vi "load_array_of_channels_xml.vi"(8 "error in":errorcluster, 11 "node in":refnum<k20>) -> (0 "error out":errorcluster, 2 "Array of DDS Channels (4)":T1=[{"Power"=FALSE, "Channel Parameters"={"Ref Clock Rate [kHz]"=1000.0, "Full Scale Output\nPower [dBm]"=0.0}, "RAM Enable"=FALSE, "RAM Dest Type"=0, "RAM Default"={"Frequency [MHz]"=0.0, "Amplitude [dBm]"=0.0, "Phase Offset [rad]"=0.0}, "Array of DDS Profiles (8)"=[], "description"=""}, {"Power"=FALSE, "Channel Parameters"={"Ref Clock Rate [kHz]"=1000.0, "Full Scale Output\nPower [dBm]"=0.0}, "RAM Enable"=FALSE, "RAM Dest Type"=0, "RAM Default"={"Frequency [MHz]"=0.0, "Amplitude [dBm]"=0.0, "Phase Offset [rad]"=0.0}, "Array of DDS Profiles (8)"=[], "description"=""}, {"Power"=FALSE, "Channel Parameters"={"Ref Clock Rate [kHz]"=1000.0, "Full Scale Output\nPower [dBm]"=0.0}, "RAM Enable"=FALSE, "RAM Dest Type"=0, "RAM Default"={"Frequency [MHz]"=0.0, "Amplitude [dBm]"=0.0, "Phase Offset [rad]"=0.0}, "Array of DDS Profiles (8)"=[], "description"=""}, {"Power"=FALSE, "Channel Parameters"={"Ref Clock Rate [kHz]"=1000.0, "Full Scale Output\nPower [dBm]"=0.0}, "RAM Enable"=FALSE, "RAM Dest Type"=0, "RAM Default"={"Frequency [MHz]"=0.0, "Amplitude [dBm]"=0.0, "Phase Offset [rad]"=0.0}, "Array of DDS Profiles (8)"=[], "description"=""}] {"Channel Parameters"."Ref Clock Rate [kHz]" min=0.0}, 3 "node":refnum<k20>)   [LabVIEW 2013, in "DDS.lvclass"]
doc: "Loads an array of DDS channels from xml. Expected format:\n\n<channel>\n<Power>%b</Power>\n<ChannelParameters.RefClockRate units=\"kHz\">%f</ChannelParameters.RefClockRate>\n<ChannelParameters.FullScaleOutputPower units=\"dBm\">%f</ChannelParameters.FullScaleOutputPower>\n<RAMEnable>%b</RAMEnable>\n<RAMDestType>%u</RAMDestType>\n<RAMDefault.Frequency units=\"MHz\">%s</RAMDefault.Frequency>\n<RAMDefault.Amplitude units=\"dBm\">%s</RAMDefault.Amplitude>\n<RAMDefault.Phase units=\"rad\">%s</RAMDefault.Phase>\n<ArrayOfDDSProfiles>\n\n<profile>\n<SingleTone.Frequency units=\"MHz\">%s</SingleTone.Frequency>\n<SingleTone.Amplitude units=\"dBm\">%s</SingleTone.Amplitude>\n<SingleTone.Phase units=\"rad\">%s</SingleTone.Phase>\n<RAMMode>%u</RAMMode>\n<ZeroCrossing>%b</ZeroCrossing>\n<NoDwellHigh>%b</NoDwellHigh>\n<FunctionOrStatic>%b</FunctionOrStatic>\n<RAMFunctionSettings>%s</RAMFunctionSettings>\n<RAMStaticArray>%s</RAMStaticArray>\n</profile>\n\n</ArrayOfDDSProfiles>\n</channel>\n\nMTL 2012 Dec 31"
uses:
  DDS.lvclass
  DDS drivers v3/array_of_DDS_channels.ctl
  DDS drivers v3/DDS_channel.ctl
  DDS drivers v3/array_of_DDS_profiles.ctl
  DDS drivers v3/DDS_profile.ctl
  DDS drivers v3/DDS RAM mode.ctl
  <vilib>/xml/Close Reference(Node).vi
  <resource>/objmgr/DOMUserDefRef.rc
  <vilib>/xml/NI_XML.lvlib
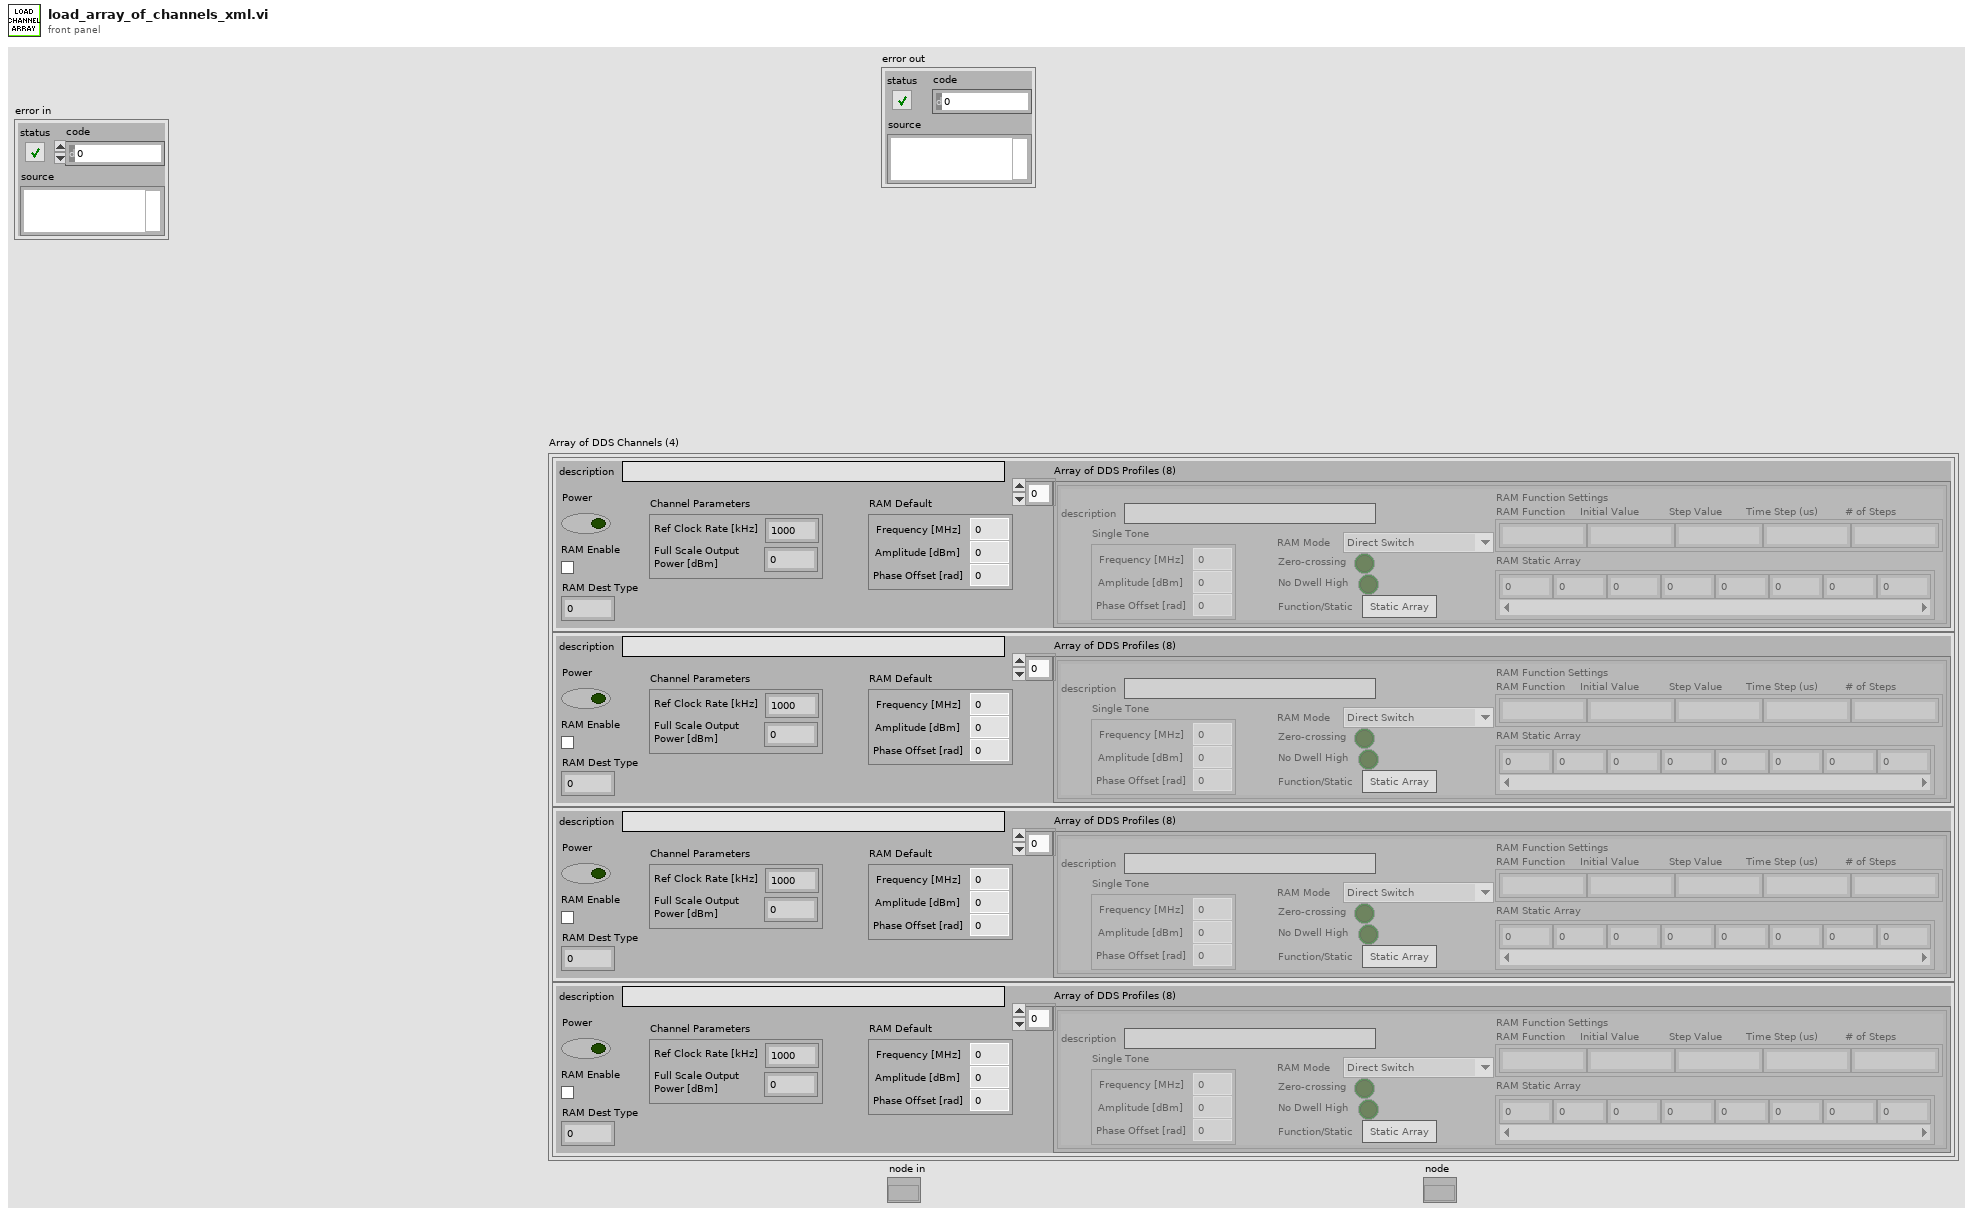
[diagram p1: front panel]
types:
  T1 = typedef "DDS.lvclass/array_of_DDS_channels.ctl" = T2[]
  T2 = typedef "DDS.lvclass/DDS_channel.ctl" = cluster{"Power":bool, "Channel Parameters":cluster{"Ref Clock Rate [kHz]":dbl, "Full Scale Output\nPower [dBm]":dbl}, "RAM Enable":bool, "RAM Dest Type":u8, "RAM Default":cluster{"Frequency [MHz]":dbl, "Amplitude [dBm]":dbl, "Phase Offset [rad]":dbl}, "Array of DDS Profiles (8)":T3, "description":string}
  T3 = typedef "DDS.lvclass/array_of_DDS_profiles.ctl" = T4[]
  T4 = typedef "DDS_profile.ctl" = cluster{"Single Tone":cluster{"Frequency [MHz]":dbl, "Amplitude [dBm]":dbl, "Phase Offset [rad]":dbl}, "RAM Mode ":T5, "Zero-crossing":bool, "No Dwell High":bool, "Function/Static":bool, "RAM Function Settings":string[], "RAM Static Array":dbl[], "description":string}
  T5 = typedef "DDS RAM mode.ctl" = enum16{"Direct Switch", "Ramp Up", "Bidirectional Ramp", "Continuous Bidirectional Ramp", "Continuous Recirculate", "Direct Switch 2", "Direct Switch 3", "Direct Switch 4"}
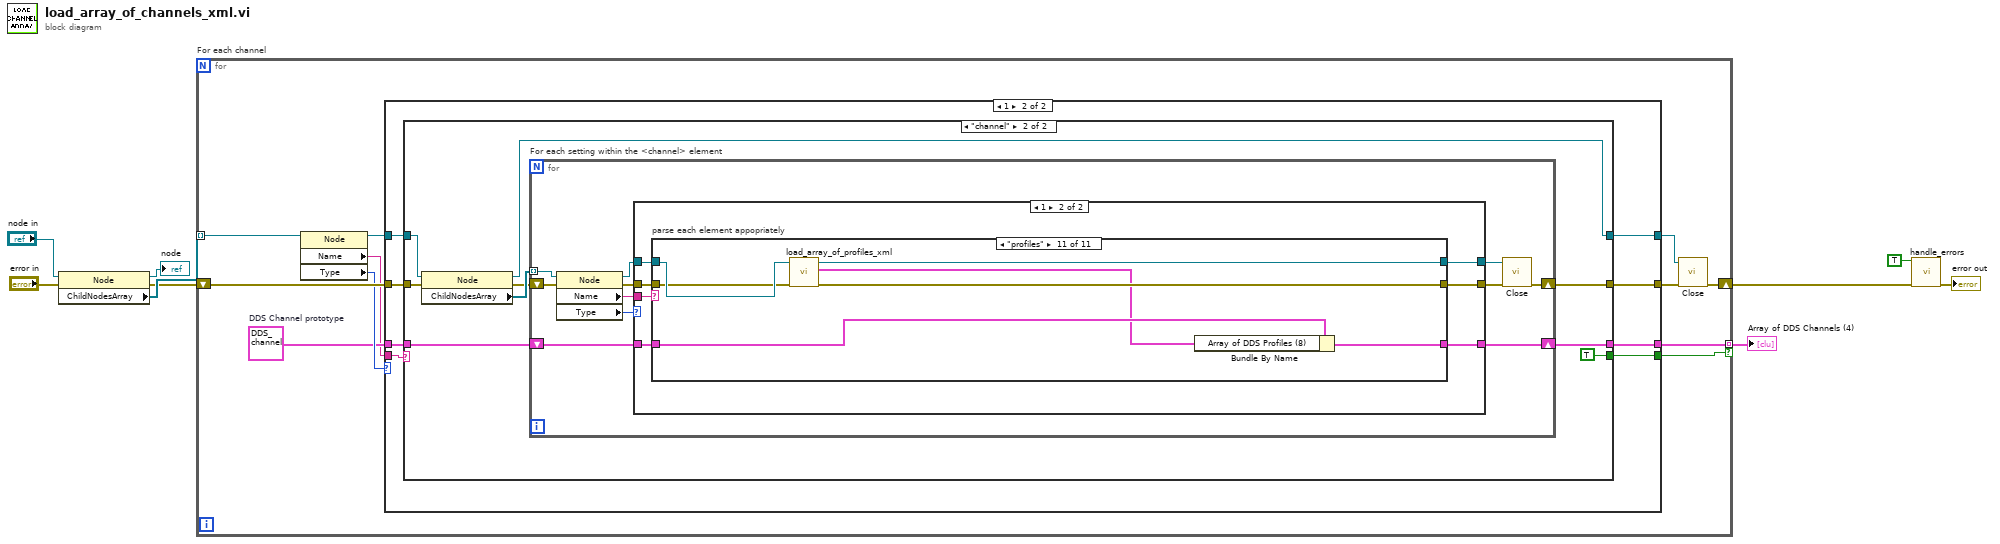
[diagram p0: block diagram]
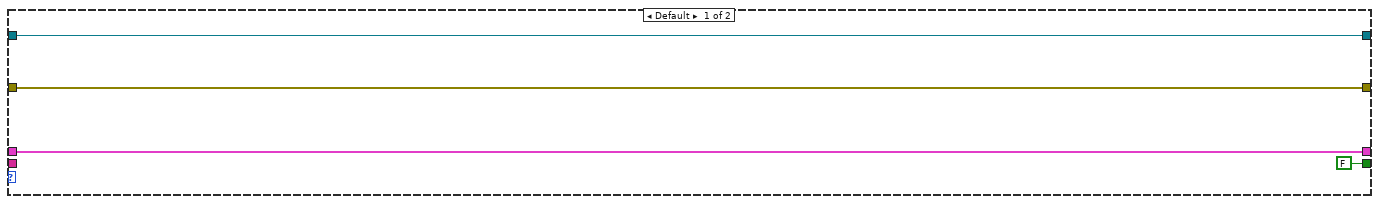
[diagram p2: hidden frame]
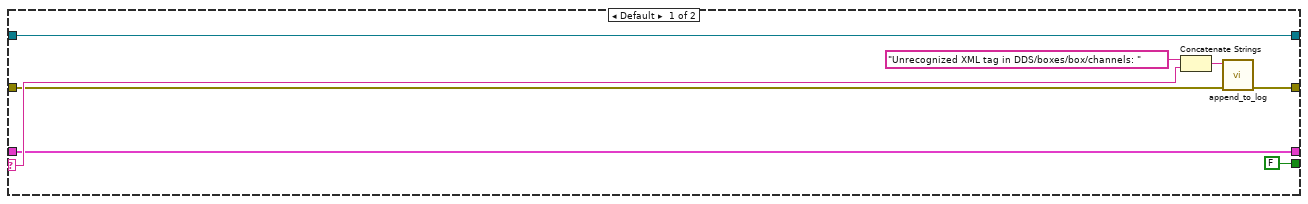
[diagram p3: hidden frame]
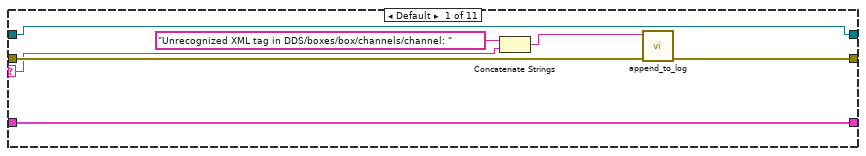
[diagram p5: hidden frame]
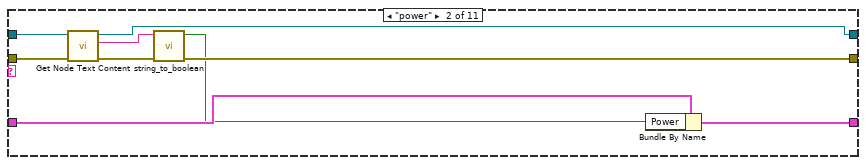
[diagram p6: hidden frame]
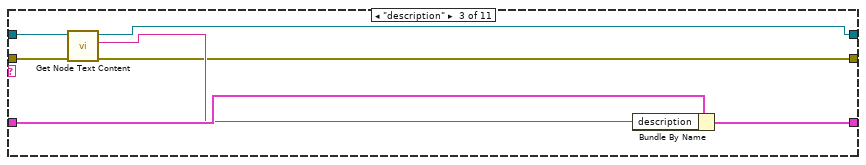
[diagram p7: hidden frame]
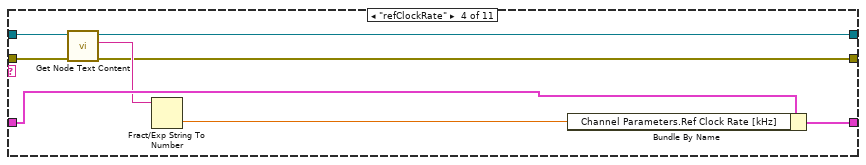
[diagram p8: hidden frame]
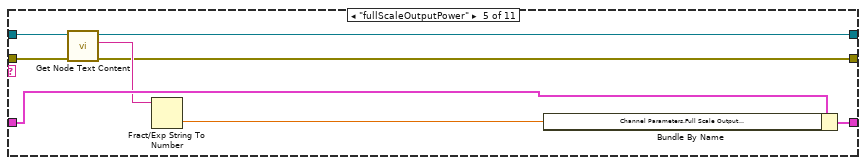
[diagram p9: hidden frame]
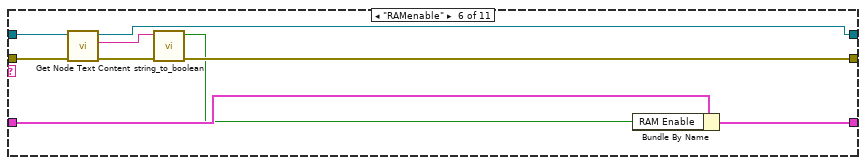
[diagram p10: hidden frame]
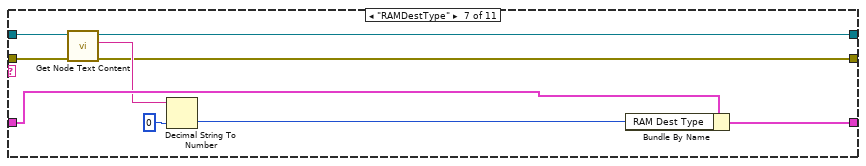
[diagram p11: hidden frame]
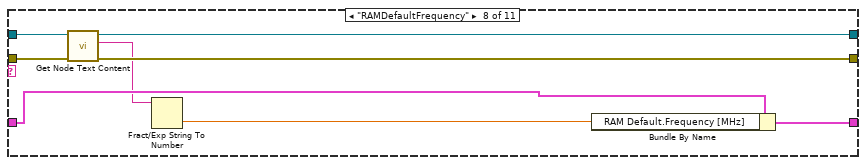
[diagram p12: hidden frame]
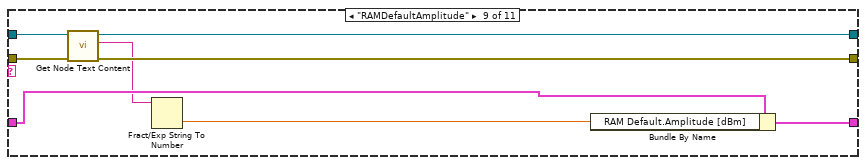
[diagram p13: hidden frame]
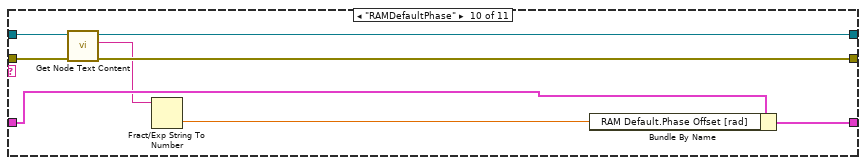
[diagram p14: hidden frame]
diagram:
  n1 = property class="Node"(reference="node in", error in="error in") -> (reference out=→"node":refnum<k20>, error out=w4:errorcluster, "ChildNodesArray"=w6:refnum<k20>[])
  n2 = for "For each channel" {
    tunnel: w6 -> [w15] mode=indexing
    shift-right: [w17] -> w2
    shift-left: w4 -> [w20]
    tunnel: [w16] -> w9 mode=indexing if=w11
    w12 = T2 {"Power"=FALSE, "Channel Parameters"={"Ref Clock Rate [kHz]"=0.0, "Full Scale Output\nPower [dBm]"=0.0}, "RAM Enable"=FALSE, "RAM Dest Type"=0, "RAM Default"={"Frequency [MHz]"=0.0, "Amplitude [dBm]"=0.0, "Phase Offset [rad]"=0.0}, "Array of DDS Profiles (8)"=[], "description"=""}  # DDS Channel prototype
    n3 = property class="Node"(reference=w15) -> (reference out=w14:refnum<k20>, "Name"=w10:string, "Type"=w13:i32)  [unwired: 1 in, 1 out]
    n4 = case shown="1" w13 {
      tunnel: w14 -> [w21 w32]
      tunnel: w20 -> [w24 w31]
      tunnel: [w21 w30] -> w19
      tunnel: [w24 w29] -> w18
      tunnel: [w23 w28] -> w16
      tunnel: w12 -> [w23 w27]
      tunnel: [FALSE w26] -> w11
      tunnel: w10 -> [_ w25]
      frame Default {
      }
      frame 1 {
        n5 = case shown="\"channel\"" w25 {
          selector: w25 -> [w38 _]
          tunnel: w32 -> [w34 w49]
          tunnel: w31 -> [w36 w48]
          tunnel: [w34 w45] -> w30
          tunnel: [w35 w44] -> w29
          tunnel: [w37 w43] -> w28
          tunnel: w27 -> [w37 w42]
          tunnel: [FALSE TRUE] -> w26
          frame Default {
            n6 = Concatenate Strings("Unrecognized XML tag in DDS/boxes/box/channels: " ("string"), w38) -> (w39:string)
            n7 = call "append_to_log.vi"("error in"=w36, "string"=w39) -> ("error out"=w35:errorcluster)  [unwired: 9 in]
          }
          frame "channel" {
            n8 = property class="Node"(reference=w49, error in=w48) -> (reference out=w45:refnum<k20>, error out=w46:errorcluster, "ChildNodesArray"=w47:refnum<k20>[])
            n9 = for "For each setting within the <channel> element" {
              tunnel: w47 -> [w60] mode=indexing
              shift-right: [w55] -> w44
              shift-left: w46 -> [w58]
              shift-right: [w51] -> w43
              shift-left: w42 -> [w52]
              n10 = property class="Node"(reference=w60, error in=w58) -> (reference out=w57:refnum<k20>, error out=w54:errorcluster, "Name"=w59:string, "Type"=w50:i32)
              n11 = case shown="1" w50 {
                tunnel: w59 -> [_ w70]
                tunnel: w57 -> [w62 w69]
                tunnel: [w62 w68] -> w56
                tunnel: w54 -> [w63 w67]
                tunnel: [w63 w66] -> w53
                tunnel: w52 -> [w61 w65]
                tunnel: [w61 w64] -> w51
                frame Default {
                }
                frame 1 {
                  n12 = case "parse each element appopriately" shown="\"profiles\"" w70 {
                    selector: w70 -> [w71 _ _ _ _ _ _ _ _ _ _]
                    tunnel: w69 -> [w77 w84 w91 w101 w107 w116 w127 w134 w141 w147 w155]
                    tunnel: [w77 w80 w89 w100 w106 w115 w119 w133 w140 w146 w153] -> w68
                    tunnel: w67 -> [w73 w83 w90 w99 w104 w114 w121 w132 w139 w148 w154]
                    tunnel: [w72 w79 w87 w94 w103 w111 w120 w131 w138 w149 w156] -> w66
                    tunnel: w65 -> [w76 w86 w93 w98 w109 w118 w126 w135 w143 w151 w158]
                    tunnel: [w76 w85 w92 w97 w108 w117 w125 w130 w142 w150 w157] -> w64
                    frame Default {
                      n13 = Concatenate Strings("Unrecognized XML tag in DDS/boxes/box/channels/channel: " ("string"), w71) -> (w74:string)
                      n14 = call "append_to_log.vi"("error in"=w73, "string"=w74) -> ("error out"=w72:errorcluster)  [unwired: 9 in]
                    }
                    frame "power" {
                      n15 = call <vilib>:"Get Node Text Content.vi"("error in (no error)"=w83, "node in"=w84) -> ("error out"=w81:errorcluster, "node text"=w82:string, "node out"=w80:refnum<k20>)  [unwired: 7 in]
                      n16 = call "string_to_boolean.vi"("error in"=w81, "string"=w82) -> ("error out"=w79:errorcluster, "boolean"=w78:bool)  [unwired: 8 in]
                      n17 = Bundle By Name(cluster=w86, "Power"=w78) -> (w85:T2)
                    }
                    frame "description" {
                      n18 = call <vilib>:"Get Node Text Content.vi"("error in (no error)"=w90, "node in"=w91) -> ("error out"=w87:errorcluster, "node text"=w88:string, "node out"=w89:refnum<k20>)  [unwired: 7 in]
                      n19 = Bundle By Name(cluster=w93, "description"=w88) -> (w92:T2)
                    }
                    frame "refClockRate" {
                      n20 = call <vilib>:"Get Node Text Content.vi"("error in (no error)"=w99, "node in"=w101) -> ("error out"=w94:errorcluster, "node text"=w96:string, "node out"=w100:refnum<k20>)  [unwired: 7 in]
                      n21 = Fract/Exp String To Number(string=w96) -> (number=w95:dbl)  [unwired: 3 in, 1 out]
                      n22 = Bundle By Name(cluster=w98, "Channel Parameters.Ref Clock Rate [kHz]"=w95) -> (w97:T2)
                    }
                    frame "fullScaleOutputPower" {
                      n23 = call <vilib>:"Get Node Text Content.vi"("error in (no error)"=w104, "node in"=w107) -> ("error out"=w103:errorcluster, "node text"=w105:string, "node out"=w106:refnum<k20>)  [unwired: 7 in]
                      n24 = Fract/Exp String To Number(string=w105) -> (number=w102:dbl)  [unwired: 3 in, 1 out]
                      n25 = Bundle By Name(cluster=w109, "Channel Parameters.Full Scale Output\nPower [dBm]"=w102) -> (w108:T2)
                    }
                    frame "RAMenable" {
                      n26 = call <vilib>:"Get Node Text Content.vi"("error in (no error)"=w114, "node in"=w116) -> ("error out"=w112:errorcluster, "node text"=w113:string, "node out"=w115:refnum<k20>)  [unwired: 7 in]
                      n27 = call "string_to_boolean.vi"("error in"=w112, "string"=w113) -> ("error out"=w111:errorcluster, "boolean"=w110:bool)  [unwired: 8 in]
                      n28 = Bundle By Name(cluster=w118, "RAM Enable"=w110) -> (w117:T2)
                    }
                    frame "RAMDestType" {
                      n29 = call <vilib>:"Get Node Text Content.vi"("error in (no error)"=w121, "node in"=w127) -> ("error out"=w120:errorcluster, "node text"=w124:string, "node out"=w119:refnum<k20>)  [unwired: 7 in]
                      n30 = Decimal String To Number(string=w124, default (0L)=u8 0 ("default (0 I32)")) -> (number=w123:u8)  [unwired: 1 in, 1 out]
                      n31 = Bundle By Name(cluster=w126, "RAM Dest Type"=w123) -> (w125:T2)
                    }
                    frame "RAMDefaultFrequency" {
                      n32 = call <vilib>:"Get Node Text Content.vi"("error in (no error)"=w132, "node in"=w134) -> ("error out"=w131:errorcluster, "node text"=w129:string, "node out"=w133:refnum<k20>)  [unwired: 7 in]
                      n33 = Fract/Exp String To Number(string=w129) -> (number=w128:dbl)  [unwired: 3 in, 1 out]
                      n34 = Bundle By Name(cluster=w135, "RAM Default.Frequency [MHz]"=w128) -> (w130:T2)
                    }
                    frame "RAMDefaultAmplitude" {
                      n35 = call <vilib>:"Get Node Text Content.vi"("error in (no error)"=w139, "node in"=w141) -> ("error out"=w138:errorcluster, "node text"=w137:string, "node out"=w140:refnum<k20>)  [unwired: 7 in]
                      n36 = Fract/Exp String To Number(string=w137) -> (number=w136:dbl)  [unwired: 3 in, 1 out]
                      n37 = Bundle By Name(cluster=w143, "RAM Default.Amplitude [dBm]"=w136) -> (w142:T2)
                    }
                    frame "RAMDefaultPhase" {
                      n38 = call <vilib>:"Get Node Text Content.vi"("error in (no error)"=w148, "node in"=w147) -> ("error out"=w149:errorcluster, "node text"=w145:string, "node out"=w146:refnum<k20>)  [unwired: 7 in]
                      n39 = Fract/Exp String To Number(string=w145) -> (number=w144:dbl)  [unwired: 3 in, 1 out]
                      n40 = Bundle By Name(cluster=w151, "RAM Default.Phase Offset [rad]"=w144) -> (w150:T2)
                    }
                    frame "profiles" {
                      n41 = call "load_array_of_profiles_xml.vi"("error in"=w154, "node in"=w155) -> ("error out"=w156:errorcluster, "Array of DDS Profiles (8)"=w152:T3, "node"=w153:refnum<k20>)  [unwired: 7 in]
                      n42 = Bundle By Name(cluster=w158, "Array of DDS Profiles (8)"=w152) -> (w157:T2)
                    }
                  }
                }
              }
              n43 = call-poly <vilib>:"Close.vi"("error in (no error)"=w53, "node"=w56) -> ("error out"=w55:errorcluster)  [unwired: 7 in]
            }
          }
        }
      }
    }
    n44 = call-poly <vilib>:"Close.vi"("error in (no error)"=w18, "node"=w19) -> ("error out"=w17:errorcluster)  [unwired: 7 in]
  }
  "Array of DDS Channels (4)" <- w9
  n45 = call "handle_errors.vi"("Exit Operation"=TRUE, "error in (no error)"=w2) -> ("error out"=→"error out":errorcluster)  [unwired: 13 in]
